vi "Cholesky Factorization.vi"   [LabVIEW 2024, in "NI_AALPro.lvlib"]
doc: "<p>Performs Cholesky factorization on a symmetric or Hermitian <a href=\"nihelplauncher://docs/csh?context=lvcore_gmath_test_positive_definite\">positive definite matrix</a>. Wire data to the <strong>A</strong> input to determine the polymorphic instance to use or <a href=\"nihelplauncher://docs/csh?context=lvcore_lvhowto_selectingdefaultinstpolyvi\">manually select</a> the instance.</p>"
uses:
  NI_AALPro.lvlib
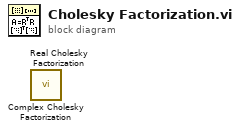
[diagram p0: block diagram]
diagram:
  n1 = call "Complex Cholesky Factorization.vi"() -> ()  [unwired: 1 in, 2 out]
  n2 = call "Real Cholesky Factorization.vi"() -> ()  [unwired: 1 in, 2 out]
